vi "ReadGlobals.vi"   [LabVIEW 2010]
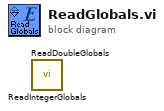
[diagram p0: block diagram]
diagram:
  n1 = call "ReadIntegerGlobals.vi"() -> ()  [unwired: 9 in, 3 out]
  n2 = call "ReadDoubleGlobals.vi"() -> ()  [unwired: 9 in, 3 out]
